vi "ValueChange.vi"(11 "left_right":bool) -> (3 "Boolean":bool)   [LabVIEW 2019, in "RT_Game.lvlib" / "Engine.lvclass"]
uses:
  Engine.lvclass
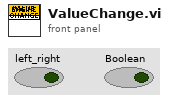
[diagram p1: front panel]
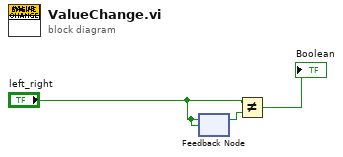
[diagram p0: block diagram]
diagram:
  n1 = feedback #1("left_right") -> (w2:bool)
  n2 = feedback-in #1("left_right") -> ()
  n3 = Not Equal?(x="left_right", y=w2) -> (x != y?=→"Boolean":bool)
